vi "92 WIO_Setting a Servo.vi"() -> ()   [LabVIEW 2024]
uses:
  <userlib>/1. Examples/_Subs/OpenDiagram/Open_XControl.xctl
  <vilib>/httpClient/POSTBuffer.vi
  <vilib>/httpClient/LabVIEWHTTPClient.lvlib
panel:
  in  "OpenDiag":refnum<vi>(xcontrol)
  out "Success":bool
  in  "Slider":dbl(slide)=161.6326530612245 scale=0.0..360.0
  out "degrees":dbl(knob) scale=0.0..40.0
  # "02 Setting a Servo\nThis code lets you control a servo on your WIO\n\nInstructions:\nInstructions:\n1. Connect up your WIO to the cloud with the phone app\n       (see http://iot.seeed.cc)\n2. Configure it to control a servo\n3. Use LabVIEW to write to the servo (enter access_token in diagram)\n       (you can get your token from the app under view API)\n4. Hit continuous run and move the slider around"
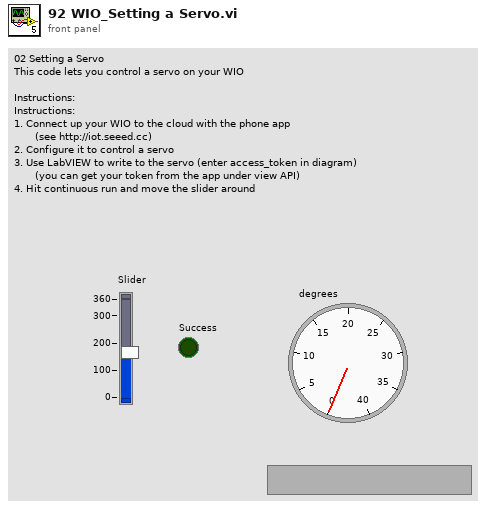
[diagram p1: front panel]
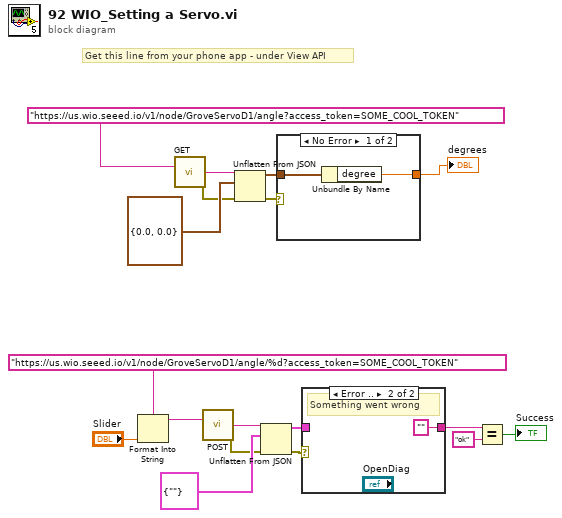
[diagram p0: block diagram]
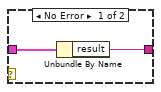
[diagram p2: hidden frame]
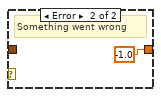
[diagram p3: hidden frame]
diagram:
  # "Get this line from your phone app - under View API"
  n1 = Format Into String(format string="https://us.wio.seeed.io/v1/node/GroveServoD1/angle/%d?access_token=SOME_COOL_TOKEN" ("url"), "Slider") -> (resulting string=w9:string)  [unwired: 2 in, 1 out]
  n2 = call <vilib>:"GET.vi"("url"="https://us.wio.seeed.io/v1/node/GroveServoD1/angle?access_token=SOME_COOL_TOKEN") -> ("body"=w17:string, "error out"=w12:errorcluster)  [unwired: 11 in, 2 out]
  n3 = call-poly <vilib>:"POST.vi"("url"=w9) -> ("body"=w7:string, "error out"=w6:errorcluster)  [unwired: 11 in, 2 out]
  n4 = Unflatten From JSON(JSON string=w17, type and defaults=cluster{"degree":dbl, "degree 2":dbl} {"degree"=0.0, "degree 2"=0.0}, error in (no error)=w12) -> (value=w15:cluster{"degree":dbl, "degree 2":dbl}, error out=w13:errorcluster)  [unwired: 4 in]
  n5 = Unflatten From JSON(JSON string=w7, type and defaults=cluster{"result":string} {"result"=""}, error in (no error)=w6) -> (value=w4:cluster{"result":string}, error out=w5:errorcluster)  [unwired: 4 in]
  n6 = case shown="No Error" w13 {
    tunnel: w15 -> [w20 _]
    tunnel: [w19 -1.0 ("temperature")] -> w14
    frame No Error {
      n7 = Unbundle By Name(w20) -> ("degree"=w19:dbl)
    }
    frame Error {
      # "Something went wrong"
    }
  }
  "degrees" <- w14
  n8 = case shown="Error .." w5 {
    tunnel: w4 -> [w23 _]
    tunnel: [w22 "" ("result")] -> w3
    frame No Error {
      n9 = Unbundle By Name(w23) -> ("result"=w22:string)
    }
    frame Error {
      # "Something went wrong"
    }
  }
  n10 = Equal?(x=w3, y="ok") -> (x = y?=→"Success":bool)
